vi "folder.volume.map.get.vi"(8 "error in (no error)":errorcluster, 11 "manager_daemon in":refnum<class "manager_daemon.lvclass">) -> (0 "error out":errorcluster, 2 "vol_ map":map{i32, map{string, i32}}(c390), 3 "manager_daemon out":refnum<class "manager_daemon.lvclass">)   [LabVIEW 2024, in "manager_daemon.lvclass"]
uses:
  manager_daemon.lvclass
  type_defs/msg--cluster.ctl
  type_defs/cmd--enum.ctl
  manager_daemon.lvclass/manager_daemon.ctl
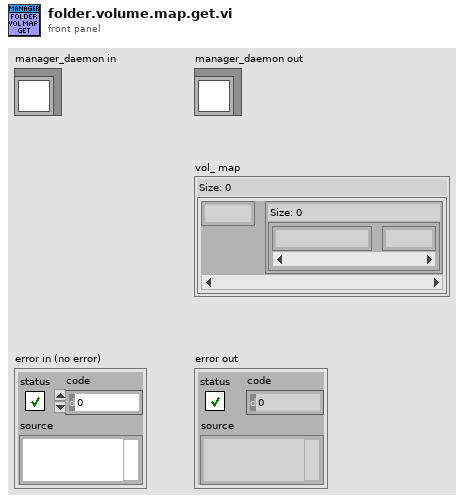
[diagram p1: front panel]
types:
  T1 = typedef "manager_daemon.lvclass/cmd--enum.ctl" = enum16{"init", "run", "load binaries", "build binaries", "save binaries", "create folder map", "display info", "apply filter", "add volume", "add issues", "add issue", "get volume", "delete volume", "delete issues", "exit"}
  T2 = typedef "manager_daemon.lvclass/msg--cluster.ctl" = cluster{"cmd":T1, "data":variant}
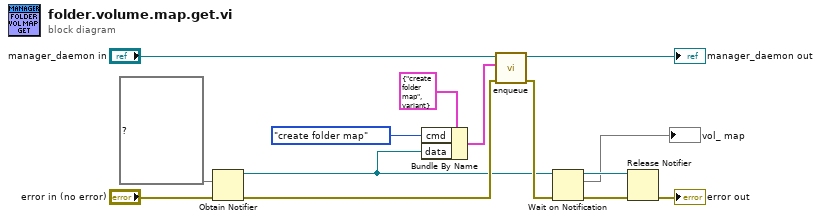
[diagram p0: block diagram]
diagram:
  n1 = Obtain Notifier(notification data type=map{i32, map{string, i32}} {} ("vol_ map"), error in (no error)="error in (no error)") -> (notifier out=w2:refnum<notifier>, error out=w3:errorcluster)  [unwired: 2 in, 1 out]
  n2 = Bundle By Name(cluster=T2 {"cmd"=enum."create folder map", "data"=variant} ("msg"), "cmd"=cmd--enum."create folder map", "data"=w2) -> (w12:T2)
  n3 = call "enqueue.vi"("error in (no error)"=w3, "msg"=w12, "manager_daemon in"="manager_daemon in") -> ("error out"=w11:errorcluster, "manager_daemon out"=→"manager_daemon out":refnum<class "manager_daemon.lvclass">)  [unwired: 7 in]
  n4 = Wait on Notification(notifier=w2, error in (no error)=w11) -> (notifier out=w9:refnum<notifier>, notification=→"vol_ map":map{i32, map{string, i32}}, error out=w8:errorcluster)  [unwired: 2 in, 1 out]
  n5 = Release Notifier(notifier=w9, error in (no error)=w8) -> (error out=→"error out":errorcluster)  [unwired: 1 in, 2 out]
